vi "Read.vi"(8 "error in (no error)":errorcluster, 11 "Simulated_Sensor in":refnum<class "Simulated_Sensor.lvclass">) -> (0 "error out":errorcluster, 2 "Numeric":dbl, 3 "Simulated_Sensor out":refnum<class "Simulated_Sensor.lvclass">)   [LabVIEW 2024, in "Sensors.lvlib" / "Simulated_Sensor.lvclass"]
uses:
  Simulated_Sensor.lvclass
  Simulated_Sensor.lvclass/Simulated_Sensor.ctl
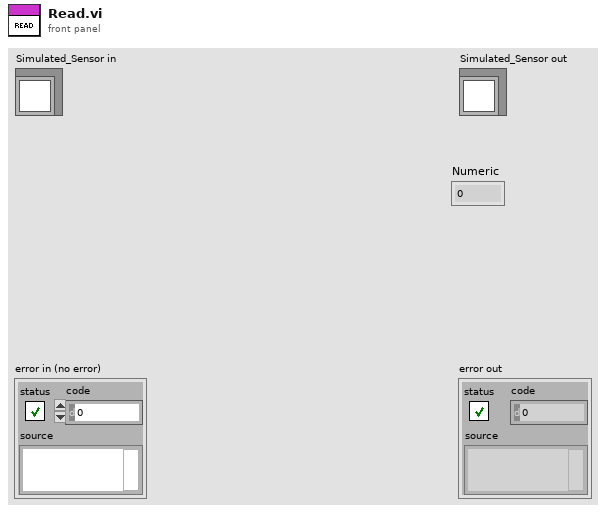
[diagram p1: front panel]
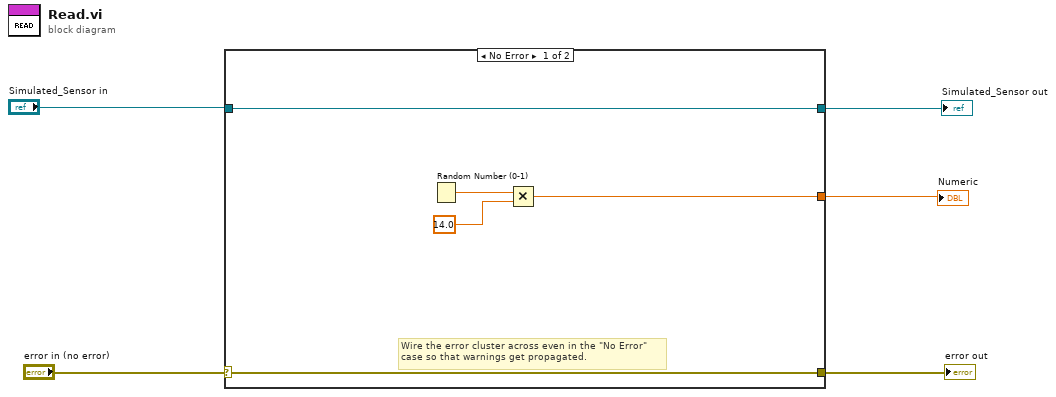
[diagram p0: block diagram]
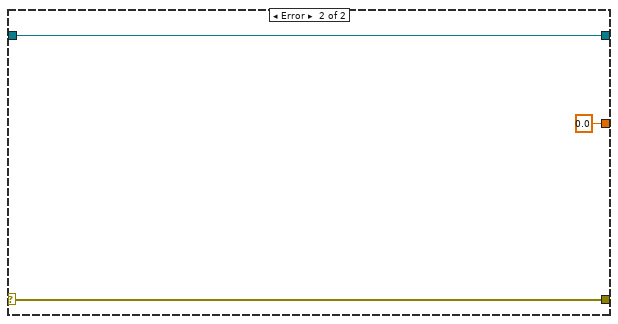
[diagram p2: hidden frame]
diagram:
  n1 = case shown="No Error" "error in (no error)" {
    selector: "error in (no error)" -> [w9 w13]
    tunnel: [w9 w13] -> w5
    tunnel: [w10 w12] -> w4
    tunnel: "Simulated_Sensor in" -> [w10 w12]
    tunnel: [w6 0.0] -> w1
    frame No Error {
      # "Wire the error cluster across even in the \"No Error\"\ncase so that warnings get propagated."
      n2 = Random Number (0-1)() -> (number: 0 to 1=w8:dbl)
      n3 = Multiply(x=w8, y=14.0) -> (x*y=w6:dbl)
    }
    frame Error {
    }
  }
  "error out" <- w5
  "Simulated_Sensor out" <- w4
  "Numeric" <- w1
